vi "Dashboard Main.vi"() -> ()   [LabVIEW 2012]
uses:
  Sally_Framework_2013/AutoEnum.ctl
  Sally_Framework_2013/LauncherPresets.ctl
  Sally_Framework_2013/AutoInstructArray.ctl
  Sally_Framework_2013/AutoInstruction.ctl
  <vilib>/event_ctls.llb/eventvkey.ctl
  DBNameEnum.ctl
  <vilib>/Utility/config.llb/Read Key (String).vi
  <vilib>/Utility/config.llb/Read Key (I32).vi
  <vilib>/Utility/config.llb/Write Key (String).vi
  <vilib>/Utility/config.llb/Write Key (I32).vi
  <vilib>/Utility/config.llb/NI_LVConfig.lvlib
panel:
  out "Battery Value":dbl(slide) scale=0.0..14.0 scale format="%#_2e"
  out "Battery":sgl(graph)
  in  "Camera Settings":T1={"Frate Rate"=30, "Compression"=30, "Size"=1} {"Frate Rate" scale=1.0..30.0; "Size" items=["640x480", "320x240", "160x120"]}
  out "Mode":T2(ring)=enum."Auto Disabled"
  out "Camera IP":string
  out "Robot IP":string
  in  "Dashboard Tab":T3(tab)
  out "ReverseDrive":bool
  in  "Use2DriveAlign":bool=TRUE
  out "DriveAlignLSRight":bool
  out "ClimbLS":bool
  in  "UseLauncherPID":bool=TRUE
  in  "UseAngleEncoder":bool=TRUE
  in  "UseLauncherEncoder":bool=TRUE
  out "LauncherAngleMatches":bool
  out "sDriveDistance":dbl
  out "Drive Loop Timing (ms)":u32
  in  "AutoEnum":T4=enum."BehindPyramid"
  out "LauncherMotorValue":dbl
  out "Version":string
  out "LauncherAngle":cluster{dbl, dbl}(knob) scale=0.0..55.0 scale format="%#2_3g"
  out "DriveAlignLSLeft":bool
  out "LauncherRPM":cluster{dbl, dbl}(knob) scale=0.0..4000.0
  in  "Disabled":T5=[{"Distance/Angle"=10.0, "Speed"=0.0, "Action"=enum."Wait", "NumFrisbees"=0}]
  in  "BehindPyramid":T5=[{"Distance/Angle"=30.0, "Speed"=2390.0, "Action"=enum."Aim", "NumFrisbees"=0}, {"Distance/Angle"=5.0, "Speed"=0.0, "Action"=enum."Wait", "NumFrisbees"=0}, {"Distance/Angle"=0.0, "Speed"=0.0, "Action"=enum."Shoot", "NumFrisbees"=4}]
  in  "CloseLeft":T5=[{"Distance/Angle"=34.0, "Speed"=2390.0, "Action"=enum."Aim", "NumFrisbees"=0}, {"Distance/Angle"=5.0, "Speed"=0.0, "Action"=enum."Wait", "NumFrisbees"=0}, {"Distance/Angle"=0.0, "Speed"=0.0, "Action"=enum."Shoot", "NumFrisbees"=4}]
  in  "CloseRight":T5=[{"Distance/Angle"=34.0, "Speed"=2390.0, "Action"=enum."Aim", "NumFrisbees"=0}, {"Distance/Angle"=5.0, "Speed"=0.0, "Action"=enum."Wait", "NumFrisbees"=0}, {"Distance/Angle"=0.0, "Speed"=0.0, "Action"=enum."Shoot", "NumFrisbees"=4}]
  in  "BackLeft":T5=[{"Distance/Angle"=29.0, "Speed"=2390.0, "Action"=enum."Aim", "NumFrisbees"=0}, {"Distance/Angle"=5.0, "Speed"=0.0, "Action"=enum."Wait", "NumFrisbees"=0}, {"Distance/Angle"=0.0, "Speed"=0.0, "Action"=enum."Shoot", "NumFrisbees"=4}]
  in  "BackRight":T5=[{"Distance/Angle"=29.0, "Speed"=2390.0, "Action"=enum."Aim", "NumFrisbees"=0}, {"Distance/Angle"=5.0, "Speed"=0.0, "Action"=enum."Wait", "NumFrisbees"=0}, {"Distance/Angle"=0.0, "Speed"=0.0, "Action"=enum."Shoot", "NumFrisbees"=4}]
  in  "BackupAuto":dbl[](array[numeric])=[2390.0, 30.0, 3.0, 4.0, 2000.0, -0.5]
  in  "UseClusterArray":bool
  in  "PullbackTol":dbl=100.0
  in  "FireTol":dbl=10.0
  in  "LauncherRPMTol":dbl=10.0
  in  "LauncherAngleTol":dbl=0.1
  in  "InitialWait (ms)":dbl=5000.0
  in  "WaitBetweenLaunch (ms)":dbl=1200.0
  in  "QSWaitBeforeFire (ms)":dbl=600.0
  in  "QSWaitBeforeRetract (ms)":dbl=100.0
  in  "AngleForwardValue":dbl=0.8
  in  "AngleBackwardValue":dbl=-0.8
  in  "HalfSpeedFactor":dbl=0.75
  in  "RPMPresets":T7={"cPresetPyramid"=2390.0, "cPresetShort"=2390.0, "cPresetMid"=1950.0, "cPresetFar"=2390.0, "cPresetClimbHigh"=0.0, "cPresetClimbLow"=0.0}
  in  "AnglePresets":T7={"cPresetPyramid"=30.0, "cPresetShort"=50.0, "cPresetMid"=51.5, "cPresetFar"=25.0, "cPresetClimbHigh"=32.0, "cPresetClimbLow"=20.0}
  in  "Slider":dbl(slide) scale=0.0..100.0 scale format="%#_3g"
  in  "On/Off":bool caption="Solenoid"
  in  "Test Name":u16(ring) items=["Select the test to run...", "Example Test", "-------------------------------", "List of tests is built in robot code.", "Replace with your own automated tests."]
  in  "Test Tree":string(tree)
  in  "Motor":cluster{"Value":dbl, "Enable":bool} {"Value" scale=-1.0..1.0 scale format="%#_3g"}
  out "Progress":T8 {"Test Progress" scale=0.0..100.0}
  in  "Rev/Fwd":cluster{"Forward":bool, "Reverse":bool}
  in  "Ring":u16(ring) items=["Auto", "Fixed indoor", "Fixed outdoor 1", "Fixed outdoor 2", "Fixed fluorescent 1", "Fixed fluorescent 2", "Hold current"]
  in  "Listbox":i32(listbox)=8
  in  "Viewer":T9(tab)
  out "Mbps":dbl format="%#.1g"
  in  "Enable":bool=TRUE
  in  "DB Camera Config":bool
  out "Mbps":bool
  out "fps":dbl format="%#.1g"
  out "Image Error Message":string="Timeout in Camera Communications"
  out "Camera Image":T10(plugin-control)
  out "Buttons 1":cluster{"1":bool, "2":bool, "3":bool}
  out "Kinect 1":cluster{"X":dbl, "Y":dbl, "Z":dbl} {"X" scale=1.0..-1.0; "Y" scale=1.0..-1.0; "Z" scale=1.0..-1.0}
  out "Buttons 2":cluster{"1":bool, "2":bool, "3":bool}
  out "Kinect 2":cluster{"X":dbl, "Y":dbl, "Z":dbl} {"X" scale=1.0..-1.0; "Y" scale=1.0..-1.0; "Z" scale=1.0..-1.0}
  out "Version":string
  out "Skeleton Picture":picture
  out "Players":i8
  out "Tree":string(tree)
  # "Drive & Motors"
  # "Robot IP:"
  # "sLauncherRPM"
  # "TargetLauncherRPM"
  # "sLauncherAngle"
  # "LauncherTargetAngle"
  # "RPM"
  # "Angle"
  # "Wait (s)"
  # "ShootNum"
  # "Time (ms)"
  # "Motor Value"
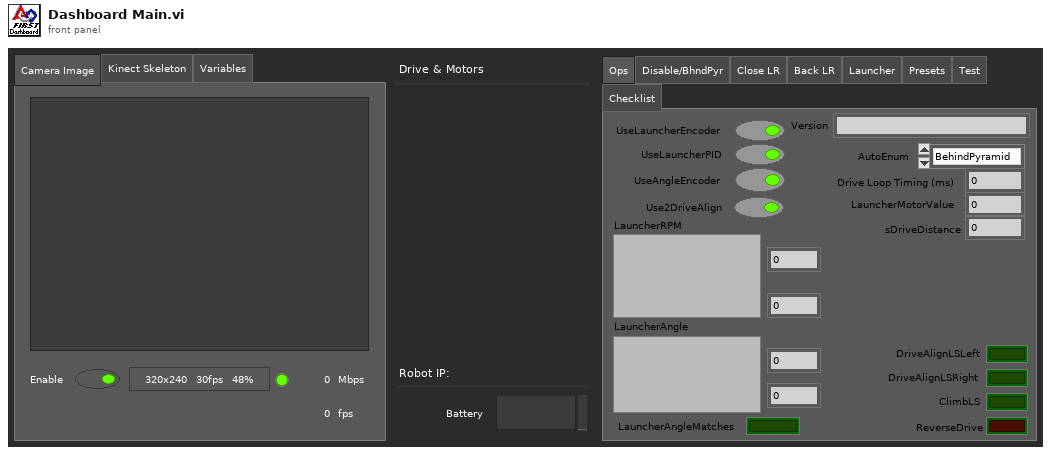
[diagram p1: front panel]
types:
  T1 = cluster{"Frate Rate":i32, "Compression":i32, "Size":u16}
  T2 = enum8{"Tele-Op Disabled", "Tele-Op Enabled", "Auto Disabled", "Auto Enabled", "Test Disabled", "Test Enabled", ""}
  T3 = enum32{"Ops", "Disable/BhndPyr", "Close LR", "Back LR", "Launcher", "Presets", "Test", "Checklist"}
  T4 = typedef "AutoEnum.ctl" = enum16{"Disabled", "BackRight", "BackLeft", "CloseRight", "CloseLeft", "BehindPyramid"}
  T5 = typedef "AutoInstructArray.ctl" = T6[]
  T6 = typedef "AutoInstruction.ctl" = cluster{"Distance/Angle":dbl, "Speed":dbl, "Action":enum16{"DriveForward", "Turn", "Aim", "Shoot", "Wait"}, "NumFrisbees":i32}
  T7 = typedef "LauncherPresets.ctl" = cluster{"cPresetPyramid":dbl, "cPresetShort":dbl, "cPresetMid":dbl, "cPresetFar":dbl, "cPresetClimbHigh":dbl, "cPresetClimbLow":dbl}
  T8 = cluster{"Test Progress":u8, "Test Progress Text":string}
  T9 = enum32{"Camera Image", "Kinect Skeleton", "Variables"}
  T10 = typedef "IMAQ Image.ctl" = refnum<image>
  T11 = typedef "Image Type" = u32
  T12 = typedef "LVBoundsTypeDef.ctl" = cluster{"Width":u32, "Height":u32}
  T13 = typedef "SkeletonTrackState.ctl" = enum32{"NotTracked", "PositionOnly", "Tracked"}
  T14 = cluster{"TrackingState":u8[], "Position":cluster{"x":sgl, "y":sgl, "z":sgl}, cluster{"x":sgl, "y":sgl, "z":sgl, sgl}[], "TrackState":T13}
  T15 = cluster{cluster{"ScaledToPercentRange":dbl, "ScaledToPercentRange":dbl, "ScaledToPercentRange":dbl}, cluster{bool, bool, bool}}[]
  T16 = cluster{cluster{"ScaledToPercentRange":dbl, "ScaledToPercentRange":dbl, "ScaledToPercentRange":dbl}, cluster{bool, bool, bool}}
  T17 = cluster{"ScaledToPercentRange":dbl, "ScaledToPercentRange":dbl, "ScaledToPercentRange":dbl}
  T18 = typedef "LVRectTypeDef.ctl" = cluster{"Left":i16, "Top":i16, "Right":i16, "Bottom":i16}
  T19 = typedef "DBNameEnum.ctl" = enum16{"AutoInstructions", "DriveLoopTime", "DriveAlignLSLeft", "DriveAlignLSRight", "Use2DriveAlign", "ClimbLS", "LauncherAngleMatches", "FrameworkVersion", "sLauncherAngle", "LauncherTargetAngle", "sLauncherRPM", "LauncherTargetRPM", "sDriveDistance", "LauncherMotorValue", "PullbackTol", "FireTol", "LauncherRPMTol", "LauncherAngleTol", "InitialWait", "WaitBetweenLaunch", "AnglePresets", "RPMPresets", "UseAngleEncoder", "UseLauncherEncoder", "UseLauncherPID", "QSWaitBeforeFire", "QSWaitBeforeRetract", "AngleForwardValue", "AngleBackwardValue", "UseClusterArray", "BackupAuto", "ReverseDriveIndicate", "HalfSpeedFactor"}
  T20 = cluster{"Competition mode":bool, "Robot Link":bool, "Autonomous":bool, "Enabled":bool, "E-Stop":bool, "Simulated":bool, "TestMode":bool, "Docked Window":bool}
  T21 = typedef "NI_LVConfig.lvlib/Config Data RefNum.ctl" = refnum<k1>
  T22 = typedef "eventvkey.ctl" = enum16{"ASCII", "Enter", "Return", "Shift", "Ctrl", "Alt", "Cmd", "Opt", "Caps", "NumLock", "Clear", "Break", "Up", "Down", "Left", "Right", "Insert", "Delete", "Home", "End", "PageUp", "PageDown", "Escape", "Help", "Pause", "ScrollLock", "F1", "F2", "F3", "F4", "F5", "F6", "F7", "F8", "F9", "F10", "F11", "F12", "F13", "F14", "F15", "F16", "F17", "F18", "F19", "F20", "F21", "F22", "F23", "F24", "Play", "VolumeUp", "VolumeDown", "Mute", "Two Byte Char"}
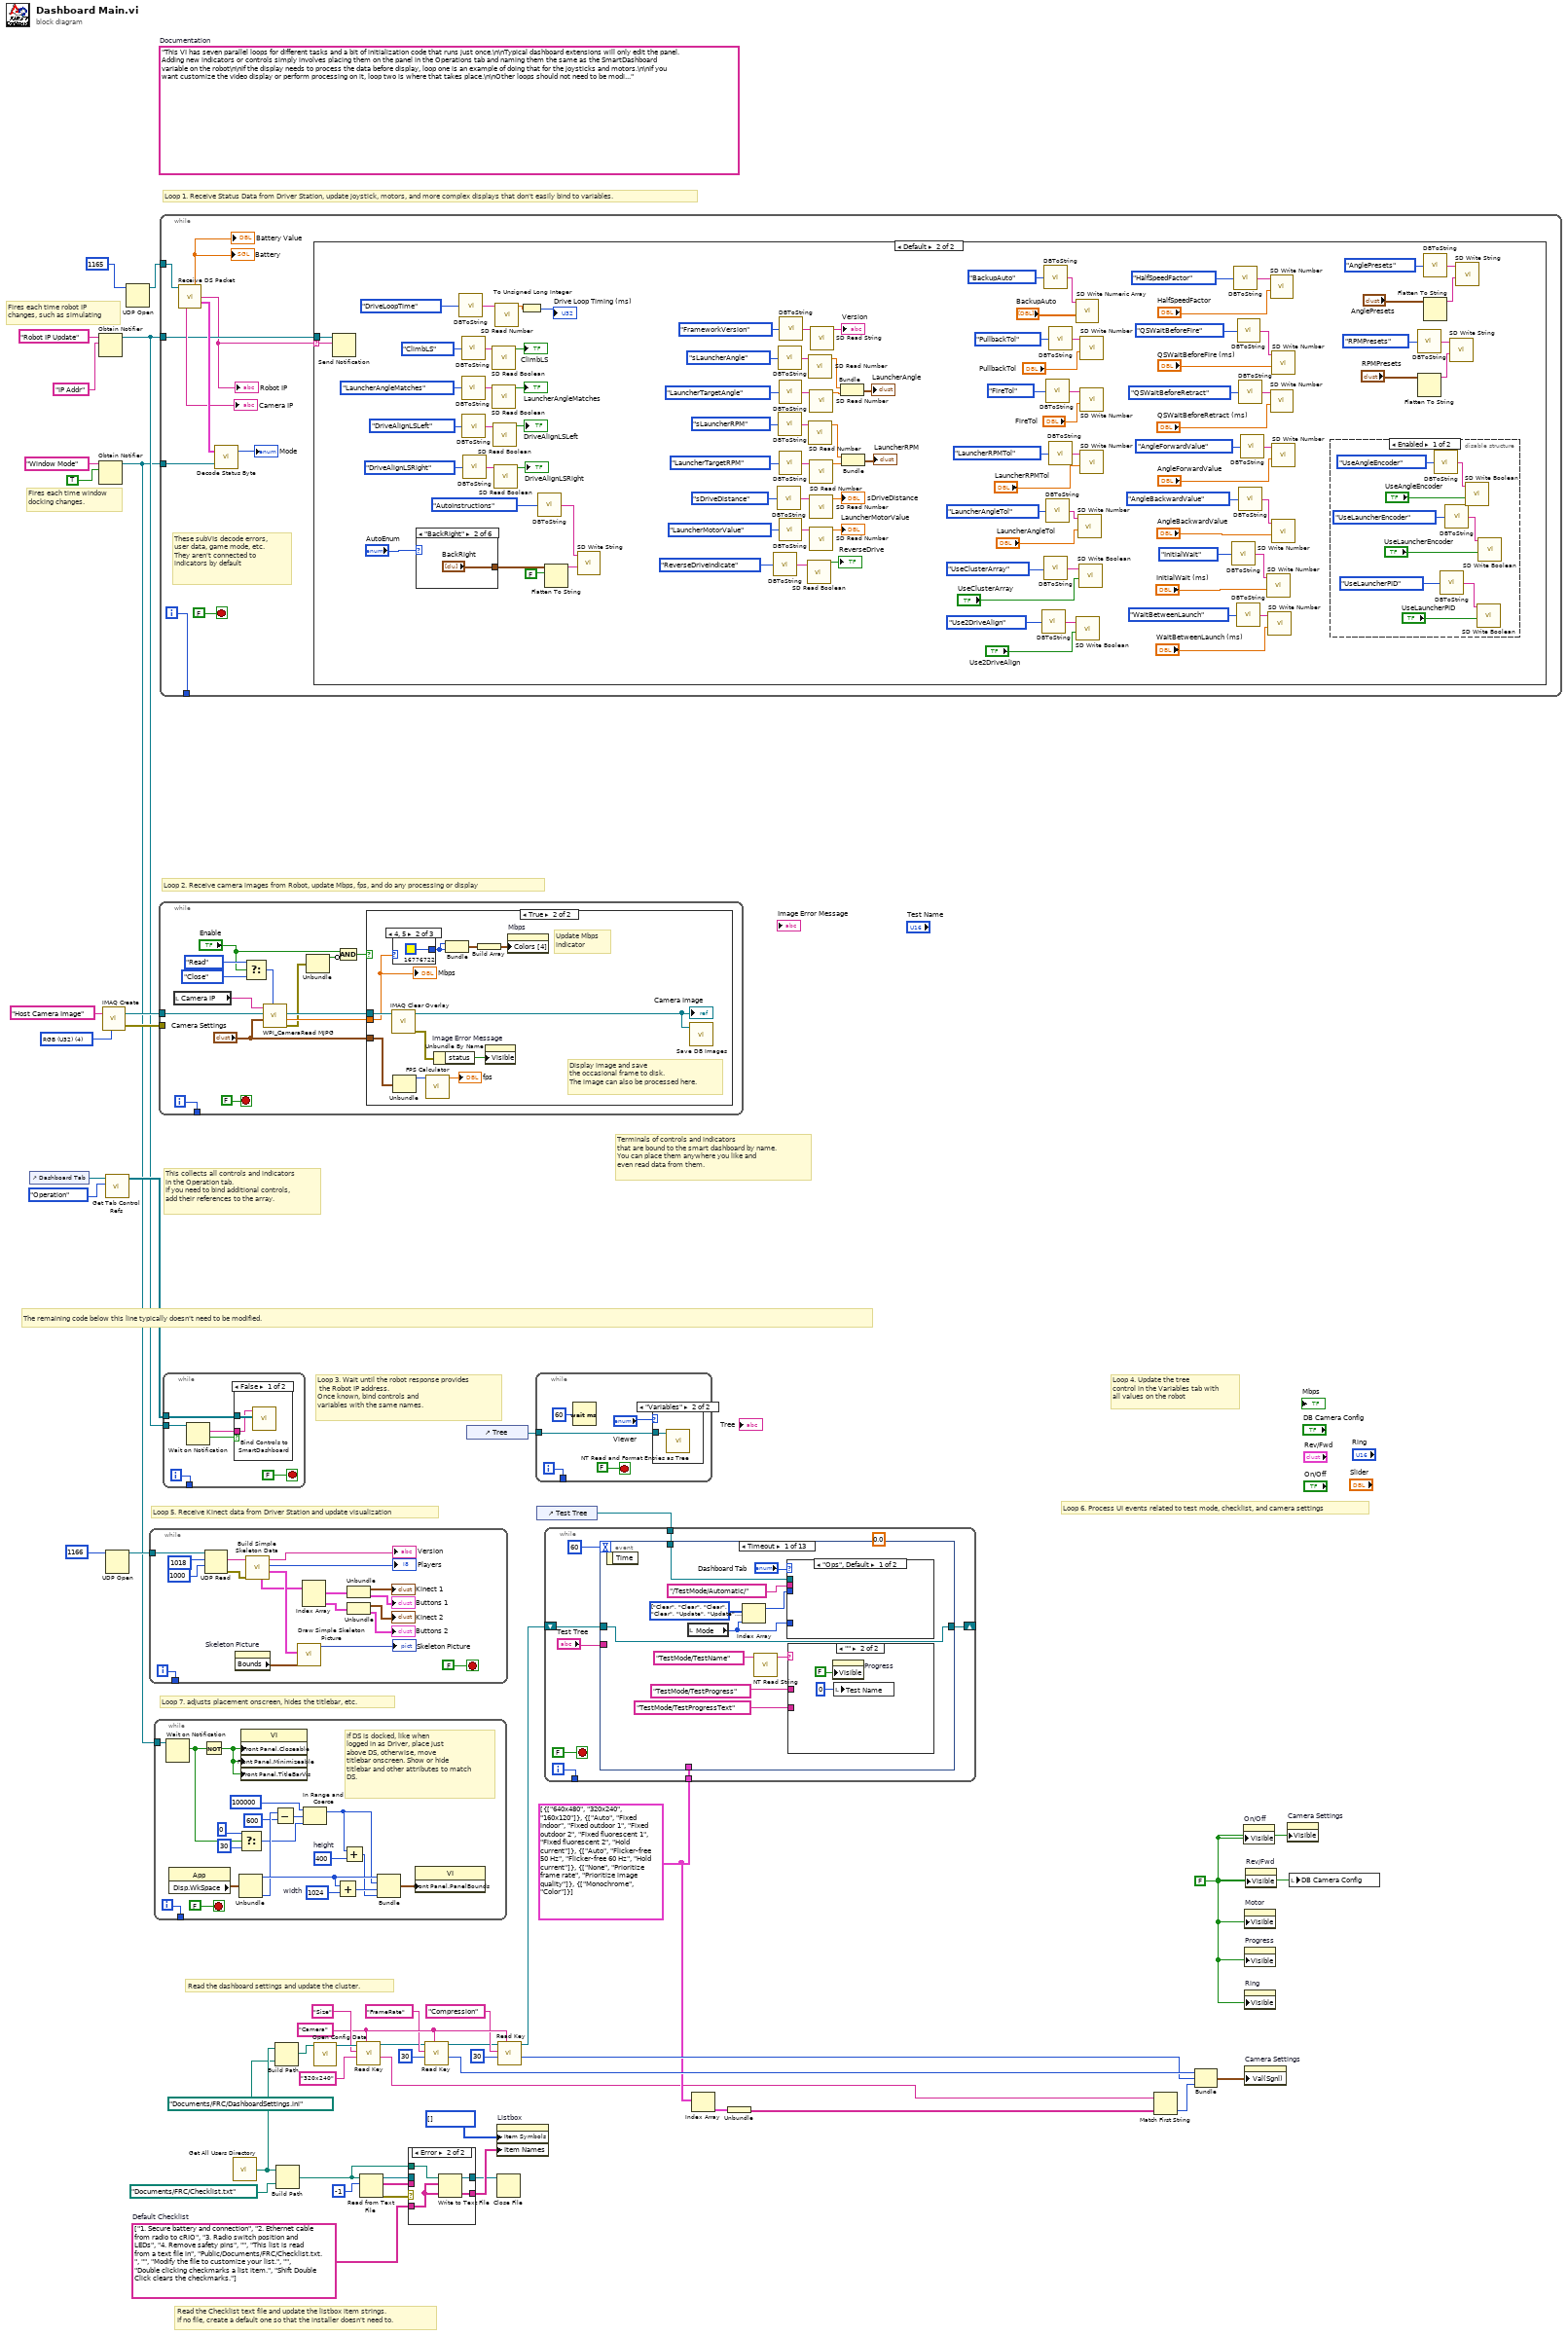
[diagram p0: block diagram]
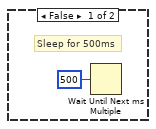
[diagram p3: hidden frame]
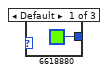
[diagram p4: hidden frame]
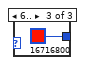
[diagram p5: hidden frame]
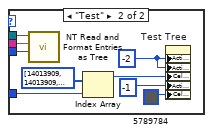
[diagram p7: hidden frame]
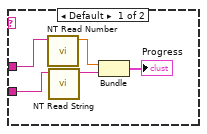
[diagram p8: hidden frame]
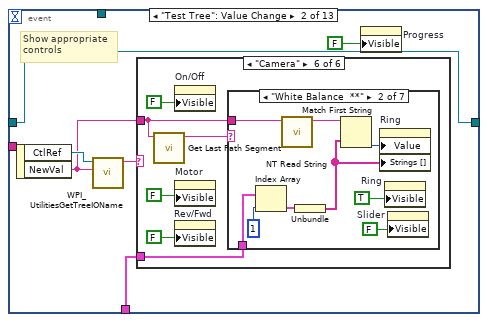
[diagram p9: hidden frame]
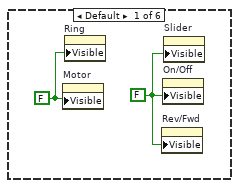
[diagram p10: hidden frame]
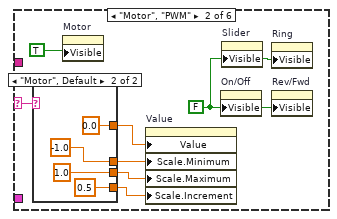
[diagram p11: hidden frame]
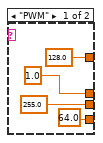
[diagram p12: hidden frame]
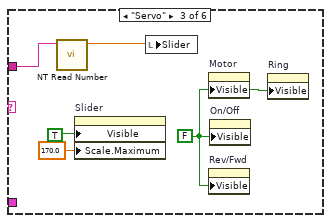
[diagram p13: hidden frame]
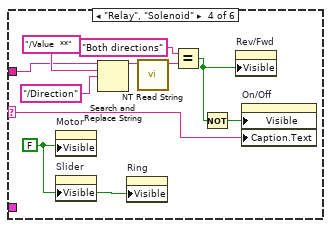
[diagram p14: hidden frame]
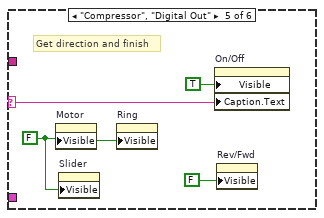
[diagram p15: hidden frame]
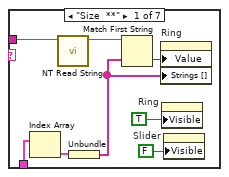
[diagram p16: hidden frame]
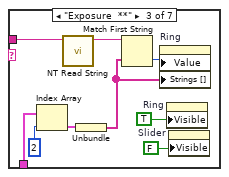
[diagram p17: hidden frame]
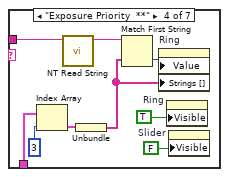
[diagram p18: hidden frame]
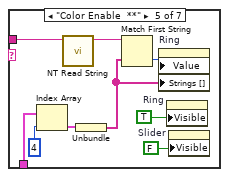
[diagram p19: hidden frame]
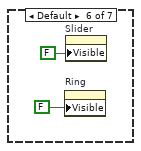
[diagram p20: hidden frame]
diagram:
  w21 = "Camera"
  w13 = cluster{string[]}[] [{["640x480", "320x240", "160x120"]}, {["Auto", "Fixed indoor", "Fixed outdoor 1", "Fixed outdoor 2", "Fixed fluorescent 1", "Fixed fluorescent 2", "Hold current"]}, {["Auto", "Flicker-free 50 Hz", "Flicker-free 60 Hz", "Hold current"]}, {["None", "Prioritize frame rate", "Prioritize image quality"]}, {["Monochrome", "Color"]}]
  w29 = string[] ["1. Secure battery and connection", "2. Ethernet cable from radio to cRIO", "3. Radio switch position and LEDs", "4. Remove safety pins", "", "This list is read from a text file in", "Public/Documents/FRC/Checklist.txt.", "", "Modify the file to customize your list.", "", "Double clicking checkmarks a list item.", "Shift Double Click clears the checkmarks."]  # Default Checklist
  w27 = FALSE ("Visible")
  (unwired) "This VI has seven parallel loops for different tasks and a bit of initialization code that runs just once.\n\nTypical dashboard extensions will only edit the panel. Adding new indicators or controls simply involves placing them on the panel in the Operations tab and naming them the same as the SmartDashboard variable on the robot\n\nIf the display needs to process the data before display, loop one is an example of doing that for the joysticks and motors.\n\nIf you want customize the video display or perform processing on it, loop two is where that takes place.\n\nOther loops should not need to be modified. They are pretty standard, and document the task they perform."  # Documentation
  w50 = T11 4 items=["Grayscale (U8)", "Grayscale (I16)", "Grayscale (SGL)", "Complex (CSG)", "RGB (U32)", "HSL (U32)", "RGB (U64)"] ("Image Type")
  # "Fires each time robot IP\nchanges, such as simulating"
  # "Fires each time window\ndocking changes."
  # "Read the Checklist text file and update the listbox item strings.\nIf no file, create a default one so that the installer doesn't need to."
  # "This collects all controls and indicators\nin the Operation tab.\nIf you need to bind additional controls,\nadd their references to the array."
  # "The remaining code below this line typically doesn't need to be modified."
  # "Loop 6. Process UI events related to test mode, checklist, and camera settings"
  # "Read the dashboard settings and update the cluster."
  # "Terminals of controls and indicators\nthat are bound to the smart dashboard by name.\nYou can place them anywhere you like and\neven read data from them."
  # "Loop 4. Update the tree\ncontrol in the Variables tab with\nall values on the robot"
  # "Loop 3. Wait until the robot response provides\n the Robot IP address.\nOnce known, bind controls and\nvariables with the same names."
  # "Loop 5. Receive Kinect data from Driver Station and update visualization"
  # "Loop 7. adjusts placement onscreen, hides the titlebar, etc."
  # "Loop 1. Receive Status Data from Driver Station, update joystick, motors, and more complex displays that don't easily bind to variables."
  # "Loop 2. Receive camera images from Robot, update Mbps, fps, and do any processing or display"
  n1 = control-ref of="Dashboard Tab"() -> (w43:refnum<vi>)
  n2 = Obtain Notifier(name (unnamed)="Robot IP Update", notification data type="IP Addr" ("name (unnamed)")) -> (notifier out=w40:refnum<notifier>)  [unwired: 2 in, 2 out]
  n3 = Obtain Notifier(name (unnamed)="Window Mode", notification data type=TRUE) -> (notifier out=w33:refnum<notifier>)  [unwired: 2 in, 2 out]
  n4 = call "IMAQ Create"("Image Name"="Host Camera Image", "Image Type"=w50) -> ("New Image"=w48:T10, "error out"=w47:errorcluster)  [unwired: 2 in, 1 out]
  n5 = call <vilib>:"Get Tab Control Refs.vi"("Page Index"=enum32{"Operation", "Test"}."Operation" ("Dashboard Tab"), "TabControl in"=w43) -> ("ControlsOnPage"=w44:refnum<vi>[])  [unwired: 9 in]
  n6 = UDP Open(11:u16 1166 ("port")) -> (port=w45:refnum<k16>)  [unwired: 2 in, 4 out]
  n7 = UDP Open(11:u16 1165 ("port")) -> (port=w51:refnum<k16>)  [unwired: 2 in, 4 out]
  n8 = while {
    tunnel: w45 -> [w69]
    tunnel: [w54] -> _
    i -> [w54]
    stop <- FALSE stop-if-true
    n9 = UDP Read(connection ID=w69, max size (548)=1018 ("bytes to read"), timeout ms (25000)=1000) -> (data out=w63:string, error out=w53:errorcluster)  [unwired: 1 in, 3 out]
    n10 = property on="Skeleton Picture" class="Pict"() -> ("Bounds"=w65:T12)  [unwired: 2 in, 2 out]
    n11 = call "Build Simple Skeleton Data.vi"("error in (no error)"=w53, "data in"=w63) -> ("Skeleton Data"=w64:T14, "NumPlayers"=→"Players":i8, "Version String"=→"Version":string, "Simple Joystick Info"=w61:T15)  [unwired: 5 in, 1 out]
    n12 = call "Draw Simple Skeleton Picture.vi"("Bounds"=w65, "Simple Skeleton"=w64) -> ("new picture out"=→"Skeleton Picture":picture)  [unwired: 9 in]
    n13 = Index Array(array=w61) -> (element #1=w60:T16, element #2=w59:T16)  [unwired: 2 in]
    n14 = Unbundle(w60) -> (→"Kinect 1":T17, →"Buttons 1":cluster{bool, bool, bool})
    n15 = Unbundle(w59) -> (→"Kinect 2":T17, →"Buttons 2":cluster{bool, bool, bool})
  }
  n16 = while {
    tunnel: w33 -> [w90]
    tunnel: [w88] -> _
    i -> [w88]
    stop <- FALSE stop-if-true
    w80 = 1024  # width
    w83 = 400  # height
    # "If DS is docked, like when\nlogged in as Driver, place just\nabove DS, otherwise, move\ntitlebar onscreen. Show or hide\ntitlebar and other attributes to match\nDS."
    n17 = Wait on Notification(notifier=w90) -> (notification=w75:bool)  [unwired: 3 in, 3 out]
    n18 = property class="App"() -> ("Disp.WkSpace"=w86:T18)  [unwired: 2 in, 2 out]
    n19 = Not(x=w75) -> (.not. x?=w89:bool)
    n20 = Unbundle(w86) -> ("Left"=w84:i16, "Bottom"=w81:i16)  [unwired: 2 out]
    n21 = Select(t=0, s=w75, f=30) -> (s? t:f=w74:i32)
    n22 = property class="VI"("Front Panel.Closeable"=w89, "Front Panel.Minimizeable"=w89, "Front Panel.TitleBarVis"=w89) -> ()  [unwired: 2 in, 2 out]
    n23 = Subtract(x=w81, y=600) -> (x-y=w78:i32)
    n24 = In Range and Coerce(upper limit=100000, x=w78, lower limit=w74) -> (coerced(x)=w72:i32)  [unwired: 1 out]
    n25 = Add(x=w84, y=w80) -> (x+y=w85:i32)
    n26 = Add(x=w72, y=w83) -> (x+y=w82:i32)
    n27 = Bundle("Left"=w84, w72, w85, w82) -> (w87:cluster{"Left":i16, i32, i32, i32})  [unwired: 1 out]
    n28 = property class="VI"("Front Panel.PanelBounds"=w87) -> ()  [unwired: 2 in, 2 out]
  }
  n29 = while {
    tunnel: w48 -> [w101]
    tunnel: w47 -> [_]
    tunnel: [w104] -> _
    i -> [w104]
    stop <- FALSE stop-if-true
    n30 = local read "Camera IP"() -> (w103:string)
    n31 = Select(t=enum16{"Read", "Reopen", "Close"}."Read" ("Operation"), s="Enable", f=enum16{"Read", "Reopen", "Close"}."Close" ("Operation")) -> (s? t:f=w96:enum16{"Read", "Reopen", "Close"})
    n32 = call <vilib>:"WPI_CameraRead MJPG.vi"("Operation"=w96, "Camera Settings"="Camera Settings", "Image"=w101, "address"=w103) -> ("error out"=w95:errorcluster, "Bandwidth (kbps)"=w99:dbl, "Image Out"=w100:T10)  [unwired: 5 in]
    n33 = Unbundle(w95) -> ("status"=w93:bool)  [unwired: 2 out]
    n34 = Compound Arithmetic op=AND("Enable", invert w93) -> (w92:bool)
    n35 = case shown="True" w92 {
      tunnel: "Camera Settings" -> [_ w108]
      tunnel: w100 -> [_ w111]
      tunnel: w99 -> [_ w110]
      frame False {
        # "Sleep for 500ms"
        n36 = Wait Until Next ms Multiple(millisecond multiple=u32 500) -> ()  [unwired: 1 out]
      }
      frame True {
        # "Display image and save\nthe occasional frame to disk.\nThe image can also be processed here."
        # "Update Mbps\nindicator"
        n37 = call "IMAQ Clear Overlay"("Image"=w111) -> ("error out"=w116:errorcluster, "Image Out"=w115:T10)  [unwired: 2 in, 7 out]
        "Camera Image" <- w115
        n38 = case shown="4, 5" w110 {
          tunnel: [u32 6618880 ("Color Box") u32 16776722 ("Color Box") u32 16716800 ("Color Box")] -> w112
          frame Default {
          }
          frame 4, 5 {
          }
          frame 6.. {
          }
        }
        n39 = Unbundle(w108) -> ("Frate Rate"=w107:i32)  [unwired: 2 out]
        n40 = call "FPS Calculator.vi"("Average Count"=w107) -> ("fps"=→"fps":dbl)  [unwired: 10 in]
        n41 = Unbundle By Name(w116) -> ("status"=w117:bool)
        n42 = Bundle("Color Box"=w112, "Color Box"=w112) -> (w114:cluster{"Color Box":u32, "Color Box":u32})  [unwired: 1 out]
        n43 = Build Array(w114) -> (w113:cluster{"Color Box":u32, "Color Box":u32}[])
        n44 = property on="Image Error Message" class="Str"("Visible"=w117) -> ()  [unwired: 2 in, 2 out]
        n45 = property on="Mbps" class="Bool (strict)"("Colors [4]"=w113) -> ()  [unwired: 2 in, 2 out]
        n46 = call "Save DB Images.vi"("Image"=w115) -> ()  [unwired: 2 in, 1 out]
        "Mbps" <- w110
      }
    }
  }
  n47 = while {
    tunnel: w51 -> [w128]
    tunnel: w40 -> [w122]
    tunnel: w33 -> [w126]
    tunnel: [w123] -> _
    i -> [w123]
    stop <- FALSE stop-if-true
    # "These subVIs decode errors, user data, game mode, etc.\nThey aren't connected to indicators by default"
    n48 = call "Receive DS Packet.vi"("Recv Socket"=w128) -> ("Battery"=→"Battery" →"Battery Value":sgl, "Robot IP Address"=w121:string, "Status"=w129:T20, "Camera IP Address"=→"Camera IP":string)  [unwired: 1 in, 10 out]
    "Robot IP" <- w121
    n49 = call "Decode Status Byte.vi"("Window Mode Notifier"=w126, "Status"=w129) -> ("Mode"=→"Mode":T2)  [unwired: 1 out]
    n50 = case shown="Default" w121 {
      selector: w121 -> [_ w229]
      tunnel: w122 -> [_ w230]
      frame "0.0.0.0" {
        # "Robot not responding, don't poll the variables"
      }
      frame Default {
        n51 = Send Notification(notification=w229, notifier=w230) -> ()  [unwired: 1 in, 2 out]
        n52 = case shown="\"BackRight\"" "AutoEnum" {
          tunnel: ["Disabled" "BackRight" "BackLeft" "CloseRight" "CloseLeft" "BehindPyramid"] -> w164
          frame "Disabled" {
          }
          frame "BackRight" {
          }
          frame "BackLeft" {
          }
          frame "CloseRight" {
          }
          frame "CloseLeft" {
          }
          frame "BehindPyramid", Default {
          }
        }
        n53 = call "DBToString.vi"("Enum"=DBNameEnum."DriveLoopTime") -> ("Refname"=w162:string)
        n54 = call "DBToString.vi"("Enum"=DBNameEnum."ClimbLS") -> ("Refname"=w170:string)
        n55 = call "DBToString.vi"("Enum"=DBNameEnum."LauncherAngleMatches") -> ("Refname"=w169:string)
        n56 = call "DBToString.vi"("Enum"=DBNameEnum."DriveAlignLSLeft") -> ("Refname"=w173:string)
        n57 = call "DBToString.vi"("Enum"=DBNameEnum."DriveAlignLSRight") -> ("Refname"=w161:string)
        n58 = call <vilib>:"SD Read Boolean.vi"("Name"=w170) -> ("Boolean"=→"ClimbLS":bool)  [unwired: 8 in, 2 out]
        n59 = call <vilib>:"SD Read Boolean.vi"("Name"=w169) -> ("Boolean"=→"LauncherAngleMatches":bool)  [unwired: 8 in, 2 out]
        n60 = call <vilib>:"SD Read Boolean.vi"("Name"=w173) -> ("Boolean"=→"DriveAlignLSLeft":bool)  [unwired: 8 in, 2 out]
        n61 = call <vilib>:"SD Read Boolean.vi"("Name"=w161) -> ("Boolean"=→"DriveAlignLSRight":bool)  [unwired: 8 in, 2 out]
        n62 = call <vilib>:"SD Read Number.vi"("Name"=w162) -> ("Numeric"=w228:dbl)  [unwired: 8 in, 2 out]
        n63 = To Unsigned Long Integer(number=w228) -> (unsigned 32bit integer=→"Drive Loop Timing (ms)":u32)
        n64 = call "DBToString.vi"("Enum"=DBNameEnum."AutoInstructions") -> ("Refname"=w167:string)
        n65 = Flatten To String(anything=w164, prepend array or string size? (T)=FALSE) -> (data string=w165:string)  [unwired: 2 in, 2 out]
        n66 = call <vilib>:"SD Write String.vi"("String"=w165, "Name"=w167) -> ()  [unwired: 8 in, 2 out]
        n67 = call "DBToString.vi"("Enum"=DBNameEnum."ReverseDriveIndicate") -> ("Refname"=w134:string)
        n68 = call "DBToString.vi"("Enum"=DBNameEnum."sDriveDistance") -> ("Refname"=w175:string)
        n69 = call "DBToString.vi"("Enum"=DBNameEnum."sLauncherAngle") -> ("Refname"=w181:string)
        n70 = call "DBToString.vi"("Enum"=DBNameEnum."sLauncherRPM") -> ("Refname"=w179:string)
        n71 = call "DBToString.vi"("Enum"=DBNameEnum."LauncherTargetAngle") -> ("Refname"=w180:string)
        n72 = call "DBToString.vi"("Enum"=DBNameEnum."LauncherTargetRPM") -> ("Refname"=w178:string)
        n73 = call "DBToString.vi"("Enum"=DBNameEnum."LauncherMotorValue") -> ("Refname"=w187:string)
        n74 = call "DBToString.vi"("Enum"=DBNameEnum."FrameworkVersion") -> ("Refname"=w177:string)
        n75 = call <vilib>:"SD Read Boolean.vi"("Name"=w134) -> ("Boolean"=→"ReverseDrive":bool)  [unwired: 8 in, 2 out]
        n76 = call <vilib>:"SD Read Number.vi"("Name"=w181) -> ("Numeric"=w214:dbl)  [unwired: 8 in, 2 out]
        n77 = call <vilib>:"SD Read Number.vi"("Name"=w179) -> ("Numeric"=w210:dbl)  [unwired: 8 in, 2 out]
        n78 = call <vilib>:"SD Read Number.vi"("Name"=w180) -> ("Numeric"=w215:dbl)  [unwired: 8 in, 2 out]
        n79 = call <vilib>:"SD Read Number.vi"("Name"=w178) -> ("Numeric"=w211:dbl)  [unwired: 8 in, 2 out]
        n80 = call <vilib>:"SD Read Number.vi"("Name"=w175) -> ("Numeric"=→"sDriveDistance":dbl)  [unwired: 8 in, 2 out]
        n81 = call <vilib>:"SD Read Number.vi"("Name"=w187) -> ("Numeric"=→"LauncherMotorValue":dbl)  [unwired: 8 in, 2 out]
        n82 = call <vilib>:"SD Read String.vi"("Name"=w177) -> ("String"=→"Version":string)  [unwired: 8 in, 2 out]
        n83 = Bundle("Numeric"=w214, "Numeric"=w215) -> (→"LauncherAngle":cluster{"Numeric":dbl, "Numeric":dbl})  [unwired: 1 in]
        n84 = Bundle("Numeric"=w210, "Numeric"=w211) -> (→"LauncherRPM":cluster{"Numeric":dbl, "Numeric":dbl})  [unwired: 1 in]
        n85 = call "DBToString.vi"("Enum"=DBNameEnum."Use2DriveAlign") -> ("Refname"=w157:string)
        n86 = call "DBToString.vi"("Enum"=DBNameEnum."BackupAuto") -> ("Refname"=w139:string)
        n87 = call "DBToString.vi"("Enum"=DBNameEnum."UseClusterArray") -> ("Refname"=w142:string)
        n88 = call "DBToString.vi"("Enum"=DBNameEnum."FireTol") -> ("Refname"=w189:string)
        n89 = call "DBToString.vi"("Enum"=DBNameEnum."LauncherAngleTol") -> ("Refname"=w191:string)
        n90 = call "DBToString.vi"("Enum"=DBNameEnum."PullbackTol") -> ("Refname"=w188:string)
        n91 = call "DBToString.vi"("Enum"=DBNameEnum."LauncherRPMTol") -> ("Refname"=w190:string)
        n92 = call <vilib>:"SD Write Numeric Array.vi"("Numeric Array"="BackupAuto", "Name"=w139) -> ()  [unwired: 8 in, 2 out]
        n93 = call <vilib>:"SD Write Boolean.vi"("Boolean"="Use2DriveAlign", "Name"=w157) -> ()  [unwired: 8 in, 2 out]
        n94 = call <vilib>:"SD Write Number.vi"("Numeric"="LauncherAngleTol", "Name"=w191) -> ()  [unwired: 8 in, 2 out]
        n95 = call <vilib>:"SD Write Boolean.vi"("Boolean"="UseClusterArray", "Name"=w142) -> ()  [unwired: 8 in, 2 out]
        n96 = call <vilib>:"SD Write Number.vi"("Numeric"="PullbackTol", "Name"=w188) -> ()  [unwired: 8 in, 2 out]
        n97 = call <vilib>:"SD Write Number.vi"("Numeric"="FireTol", "Name"=w189) -> ()  [unwired: 8 in, 2 out]
        n98 = call <vilib>:"SD Write Number.vi"("Numeric"="LauncherRPMTol", "Name"=w190) -> ()  [unwired: 8 in, 2 out]
        n99 = call "DBToString.vi"("Enum"=DBNameEnum."InitialWait") -> ("Refname"=w203:string)
        n100 = call "DBToString.vi"("Enum"=DBNameEnum."HalfSpeedFactor") -> ("Refname"=w131:string)
        n101 = call "DBToString.vi"("Enum"=DBNameEnum."WaitBetweenLaunch") -> ("Refname"=w202:string)
        n102 = call "DBToString.vi"("Enum"=DBNameEnum."QSWaitBeforeFire") -> ("Refname"=w153:string)
        n103 = call "DBToString.vi"("Enum"=DBNameEnum."QSWaitBeforeRetract") -> ("Refname"=w150:string)
        n104 = call "DBToString.vi"("Enum"=DBNameEnum."AngleBackwardValue") -> ("Refname"=w144:string)
        n105 = call "DBToString.vi"("Enum"=DBNameEnum."AngleForwardValue") -> ("Refname"=w147:string)
        n106 = call <vilib>:"SD Write Number.vi"("Numeric"="InitialWait (ms)", "Name"=w203) -> ()  [unwired: 8 in, 2 out]
        n107 = call <vilib>:"SD Write Number.vi"("Numeric"="WaitBetweenLaunch (ms)", "Name"=w202) -> ()  [unwired: 8 in, 2 out]
        n108 = call <vilib>:"SD Write Number.vi"("Numeric"="HalfSpeedFactor", "Name"=w131) -> ()  [unwired: 8 in, 2 out]
        n109 = call <vilib>:"SD Write Number.vi"("Numeric"="QSWaitBeforeRetract (ms)", "Name"=w150) -> ()  [unwired: 8 in, 2 out]
        n110 = call <vilib>:"SD Write Number.vi"("Numeric"="QSWaitBeforeFire (ms)", "Name"=w153) -> ()  [unwired: 8 in, 2 out]
        n111 = call <vilib>:"SD Write Number.vi"("Numeric"="AngleForwardValue", "Name"=w147) -> ()  [unwired: 8 in, 2 out]
        n112 = call <vilib>:"SD Write Number.vi"("Numeric"="AngleBackwardValue", "Name"=w144) -> ()  [unwired: 8 in, 2 out]
        n113 = disable-structure shown="Enabled" {
          frame Enabled {
            n114 = call "DBToString.vi"("Enum"=DBNameEnum."UseAngleEncoder") -> ("Refname"=w242:string)
            n115 = call "DBToString.vi"("Enum"=DBNameEnum."UseLauncherPID") -> ("Refname"=w237:string)
            n116 = call "DBToString.vi"("Enum"=DBNameEnum."UseLauncherEncoder") -> ("Refname"=w238:string)
            n117 = call <vilib>:"SD Write Boolean.vi"("Boolean"="UseAngleEncoder", "Name"=w242) -> ()  [unwired: 8 in, 2 out]
            n118 = call <vilib>:"SD Write Boolean.vi"("Boolean"="UseLauncherPID", "Name"=w237) -> ()  [unwired: 8 in, 2 out]
            n119 = call <vilib>:"SD Write Boolean.vi"("Boolean"="UseLauncherEncoder", "Name"=w238) -> ()  [unwired: 8 in, 2 out]
          }
          frame Disabled {
          }
        }
        n120 = call "DBToString.vi"("Enum"=DBNameEnum."RPMPresets") -> ("Refname"=w198:string)
        n121 = Flatten To String(anything="RPMPresets") -> (data string=w222:string)  [unwired: 3 in, 2 out]
        n122 = call "DBToString.vi"("Enum"=DBNameEnum."AnglePresets") -> ("Refname"=w197:string)
        n123 = Flatten To String(anything="AnglePresets") -> (data string=w223:string)  [unwired: 3 in, 2 out]
        n124 = call <vilib>:"SD Write String.vi"("String"=w222, "Name"=w198) -> ()  [unwired: 8 in, 2 out]
        n125 = call <vilib>:"SD Write String.vi"("String"=w223, "Name"=w197) -> ()  [unwired: 8 in, 2 out]
      }
    }
  }
  n126 = while {
    tunnel: w44 -> [w251]
    tunnel: w40 -> [w248]
    tunnel: [w246] -> _
    i -> [w246]
    stop <- FALSE stop-if-true
    n127 = Wait on Notification(notifier=w248) -> (notification=w247:string, timed out?=w249:bool)  [unwired: 3 in, 2 out]
    n128 = case shown="False" w249 {
      tunnel: w251 -> [w253 _]
      tunnel: w247 -> [w252 _]
      frame False {
        n129 = call <vilib>:"Bind Controls to SmartDashboard.vi"("Bound Control Refs"=w253, "Server IP Address"=w252) -> ()  [unwired: 10 in]
      }
      frame True {
      }
    }
  }
  n130 = call "Get All Users Directory.vi"() -> ("All User Path"=w26:path)
  n131 = Build Path(base path=w26, name or relative path=path "Documents/FRC/DashboardSettings.ini") -> (appended path=w25:path)
  n132 = Build Path(base path=w26, name or relative path=path "Documents/FRC/Checklist.txt") -> (appended path=w30:path)
  n133 = call <vilib>:"Open Config Data.vi"("configuration file path"=w25) -> ("refnum"=w24:T21)  [unwired: 8 in, 2 out]
  n134 = call-poly <vilib>:"Read Key.vi"("section"=w21, "default value"="320x240", "key"="Size", "refnum"=w24) -> ("value"=w11:string, "refnum out"=w6:T21)  [unwired: 2 in, 4 out]
  n135 = Read from Text File(file (use dialog)=w30, count=-1 ("timeout ms (25000)")) -> (refnum out=w8:refnum<file>, text=w31:string[], error out=w32:errorcluster)  [unwired: 2 in, 1 out]
  n136 = case shown="Error" w32 {
    tunnel: w31 -> [w255 _]
    tunnel: [w255 w257] -> w28
    tunnel: w29 -> [_ w257]
    tunnel: w30 -> [_ w258]
    tunnel: [w254 w256] -> w7
    tunnel: w8 -> [w254 _]
    frame No Error {
    }
    frame Error {
      n137 = Write to Text File(file (use dialog)=w258, text=w257) -> (refnum out=w256:refnum<file>)  [unwired: 2 in, 2 out]
    }
  }
  n138 = call-poly <vilib>:"Read Key.vi"("section"=w21, "default value"=30, "key"="FrameRate", "refnum"=w6) -> ("value"=w16:i32, "refnum out"=w5:T21)  [unwired: 1 in, 5 out]
  n139 = control-ref of="Tree"() -> (w2:refnum<vi>)
  n140 = property on="Listbox" class="LstBox (strict)"("Item Symbols"=i32[] [], "Item Names"=w28) -> ()  [unwired: 2 in, 2 out]
  n141 = Close File(refnum=w7) -> ()  [unwired: 1 in, 2 out]
  n142 = call-poly <vilib>:"Read Key.vi"("section"=w21, "default value"=30, "key"="Compression", "refnum"=w5) -> ("value"=w15:i32, "refnum out"=w3:T21)  [unwired: 1 in, 5 out]
  n143 = while {
    tunnel: [w260] -> _
    tunnel: w2 -> [w259]
    i -> [w260]
    stop <- FALSE stop-if-true
    n144 = Wait (ms)(milliseconds to wait=u32 60) -> ()  [unwired: 1 out]
    n145 = case shown="\"Variables\"" "Viewer" {
      tunnel: w259 -> [_ w264]
      frame Default {
      }
      frame "Variables" {
        n146 = call <vilib>:"NT Read and Format Entries as Tree.vi"("Tree Refnum"=w264) -> ()  [unwired: 9 in, 2 out]
      }
    }
  }
  n147 = control-ref of="Test Tree"() -> (w1:refnum<vi>)
  n148 = while {
    tunnel: w13 -> [w269]
    shift-right: [w268] -> _
    shift-left: w3 -> [w267]
    tunnel: [w266] -> _
    tunnel: w1 -> [w265]
    i -> [w266]
    stop <- FALSE stop-if-true
    (unwired) 0.0 ("Meter")
    n149 = event shown="[0] Timeout" {
      selector: _ -> [_ _ _ _ _ _ _ _ _ _ _ _ _]
      dyn-events: _ -> [_ _ _ _ _ _ _ _ _ _ _ _ _]
      timeout: u32 60 ("milliseconds to wait") -> [_ _ _ _ _ _ _ _ _ _ _ _ _]
      tunnel: w265 -> [w279 _ _ _ _ _ _ _ _ _ _ _ _]
      tunnel: "Test Tree" -> [_ _ _ _ _ _ _ _ w473 w481 w483 w487 w495]
      tunnel: w269 -> [_ w301 _ _ _ _ w437 w467 _ _ _ _ _]
      tunnel: [w273 w300 _ w403 w411 w423 w436 w460 w472 w479 w482 w486 w494] -> w268
      tunnel: w267 -> [w273 w300 _ w403 w411 w423 w435 w460 w472 w479 w482 w486 w494]
      event Timeout {
        w278 = enum16{"Update", "Clear"}[] [enum."Clear", enum."Clear", enum."Clear", enum."Clear", enum."Update", enum."Update", enum."Clear"] items=["Update", "Clear"]
        n150 = event-data() -> ()  [unwired: 1 in, 1 out]
        n151 = local read "Mode"() -> (w276:T2)
        n152 = Index Array(array=w278, index=w276) -> (element=w277:enum16{"Update", "Clear"})
        n153 = call <vilib>:"NT Read String.vi"("Name"="TestMode/TestName") -> ("String"=w282:string)  [unwired: 9 in, 1 out]
        n154 = case shown="\"Ops\", Default" "Dashboard Tab" {
          tunnel: w279 -> [_ w292]
          tunnel: "/TestMode/Automatic/" ("Name Pattern") -> [_ w291]
          tunnel: w277 -> [_ w290]
          tunnel: w276 -> [_ w288]
          frame "Ops", Default {
          }
          frame "Test" {
            w287 = -2 ("Active Item:Row Number")
            n155 = call <vilib>:"NT Read and Format Entries as Tree.vi"("Operation"=w290, "Name Pattern"=w291, "Tree Refnum"=w292) -> ()  [unwired: 7 in, 2 out]
            n156 = Index Array(array=u32[] [14013909, 14013909, 14013909, 14013909, 14013909, 16777215, 14013909], index=w288) -> (element=w286:u32)
            n157 = property on="Test Tree" class="Tree (strict)"("Active Item Row Number"=w287, "ActiveColNum"=w287, "CellBG"=w286, "Active Item Row Number"=-1 ("Active Item:Row Number"), "CellBG"=u32 5789784 ("Color Box")) -> ()  [unwired: 2 in, 2 out]
          }
        }
        n158 = case shown="\"\"" w282 {
          tunnel: "TestMode/TestProgress" ("Name") -> [w294 _]
          tunnel: "TestMode/TestProgressText" ("Name") -> [w293 _]
          frame Default {
            n159 = call <vilib>:"NT Read Number.vi"("Name"=w294) -> ("Numeric"=w295:dbl)  [unwired: 9 in, 1 out]
            n160 = call <vilib>:"NT Read String.vi"("Name"=w293) -> ("String"=w296:string)  [unwired: 9 in, 1 out]
            n161 = Bundle("Numeric"=w295, "String"=w296) -> (→"Progress":cluster{"Numeric":dbl, "String":string})  [unwired: 1 in]
          }
          frame "" {
            n162 = property on="Progress" class="Clust (strict)"("Visible"=FALSE) -> ()  [unwired: 2 in, 2 out]
            n163 = local write "Test Name"(u16 0) -> ()
          }
        }
      }
      event "Test Tree": Value Change {
        # "Show appropriate\ncontrols"
        n164 = event-data() -> ("CtlRef"=w304:refnum<vi>, "NewVal"=w302:string)  [unwired: 1 in]
        n165 = call <vilib>:"WPI_UtilitiesGetTreeIOName.vi"("NewVal"=w302, "TreeControl in"=w304) -> ("I/O Name"=w305:string)  [unwired: 9 in]
        n166 = case shown="\"Camera\"" w305 {
          selector: w305 -> [_ w312 _ w330 w339 _]
          tunnel: w302 -> [_ _ w327 w329 _ w346]
          tunnel: w301 -> [_ _ _ _ _ w345]
          frame Default {
            w307 = FALSE ("Visible")
            w306 = FALSE ("Visible")
            n167 = property on="Motor" class="Clust (strict)"("Visible"=w306) -> ()  [unwired: 2 in, 2 out]
            n168 = property on="Ring" class="Ring (strict)"("Visible"=w306) -> ()  [unwired: 2 in, 2 out]
            n169 = property on="Rev/Fwd" class="Clust (strict)"("Visible"=w307) -> ()  [unwired: 2 in, 2 out]
            n170 = property on="On/Off" class="Bool (strict)"("Visible"=w307) -> ()  [unwired: 2 in, 2 out]
            n171 = property on="Slider" class="Slide (strict)"("Visible"=w307) -> ()  [unwired: 2 in, 2 out]
          }
          frame "Motor", "PWM" {
            w313 = FALSE ("Visible")
            n172 = case shown="\"Motor\", Default" w312 {
              tunnel: [1.0 ("Value") -1.0 ("Value")] -> w311
              tunnel: [255.0 ("Value") 1.0 ("Value")] -> w310
              tunnel: [128.0 ("Value") 0.0 ("Value")] -> w309
              tunnel: [64.0 ("Value") 0.5 ("Value")] -> w308
              frame "PWM" {
              }
              frame "Motor", Default {
              }
            }
            n173 = property on="Motor" class="Clust (strict)"("Visible"=TRUE) -> ()  [unwired: 2 in, 2 out]
            n174 = property on="Value" class="Slide (strict)"("Value"=w309, "Scale.Minimum"=w311, "Scale.Maximum"=w310, "Scale.Increment"=w308) -> ()  [unwired: 2 in, 2 out]
            n175 = property on="On/Off" class="Bool (strict)"("Visible"=w313) -> ()  [unwired: 2 in, 2 out]
            n176 = property on="Slider" class="Slide (strict)"("Visible"=w313) -> ()  [unwired: 2 in, 2 out]
            n177 = property on="Ring" class="Ring (strict)"("Visible"=w313) -> ()  [unwired: 2 in, 2 out]
            n178 = property on="Rev/Fwd" class="Clust (strict)"("Visible"=w313) -> ()  [unwired: 2 in, 2 out]
          }
          frame "Servo" {
            w325 = FALSE ("Visible")
            n179 = call <vilib>:"NT Read Number.vi"("Name"=w327) -> ("Numeric"=w326:dbl)  [unwired: 9 in, 1 out]
            n180 = property on="Slider" class="Slide (strict)"("Visible"=TRUE, "Scale.Maximum"=170.0 ("Scale.Range:Maximum")) -> ()  [unwired: 2 in, 2 out]
            n181 = local write "Slider"(w326) -> ()
            n182 = property on="Motor" class="Clust (strict)"("Visible"=w325) -> ()  [unwired: 2 in, 2 out]
            n183 = property on="Rev/Fwd" class="Clust (strict)"("Visible"=w325) -> ()  [unwired: 2 in, 2 out]
            n184 = property on="On/Off" class="Bool (strict)"("Visible"=w325) -> ()  [unwired: 2 in, 2 out]
            n185 = property on="Ring" class="Ring (strict)"("Visible"=w325) -> ()  [unwired: 2 in, 2 out]
          }
          frame "Relay", "Solenoid" {
            w328 = FALSE ("Visible")
            n186 = property on="Motor" class="Clust (strict)"("Visible"=w328) -> ()  [unwired: 2 in, 2 out]
            n187 = property on="Slider" class="Slide (strict)"("Visible"=w328) -> ()  [unwired: 2 in, 2 out]
            n188 = Search and Replace String(input string=w329, search string="/Value  **", replace string="/Direction") -> (result string=w335:string)  [unwired: 5 in, 3 out]
            n189 = property on="Ring" class="Ring (strict)"("Visible"=w328) -> ()  [unwired: 2 in, 2 out]
            n190 = call <vilib>:"NT Read String.vi"("Name"=w335) -> ("String"=w333:string)  [unwired: 9 in, 1 out]
            n191 = Equal?(x="Both directions", y=w333) -> (x = y?=w331:bool)
            n192 = Not(x=w331) -> (.not. x?=w332:bool)
            n193 = property on="Rev/Fwd" class="Clust (strict)"("Visible"=w331) -> ()  [unwired: 2 in, 2 out]
            n194 = property on="On/Off" class="Bool (strict)"("Visible"=w332, "Caption.Text"=w330) -> ()  [unwired: 2 in, 2 out]
          }
          frame "Compressor", "Digital Out" {
            w338 = FALSE ("Visible")
            # "Get direction and finish"
            n195 = property on="Motor" class="Clust (strict)"("Visible"=w338) -> ()  [unwired: 2 in, 2 out]
            n196 = property on="Slider" class="Slide (strict)"("Visible"=w338) -> ()  [unwired: 2 in, 2 out]
            n197 = property on="Ring" class="Ring (strict)"("Visible"=w338) -> ()  [unwired: 2 in, 2 out]
            n198 = property on="On/Off" class="Bool (strict)"("Visible"=TRUE, "Caption.Text"=w339) -> ()  [unwired: 2 in, 2 out]
            n199 = property on="Rev/Fwd" class="Clust (strict)"("Visible"=FALSE) -> ()  [unwired: 2 in, 2 out]
          }
          frame "Camera" {
            n200 = call <vilib>:"Get Last Path Segment.vi"("String in"=w346) -> ("String out"=w347:string)  [unwired: 10 in]
            n201 = property on="On/Off" class="Bool (strict)"("Visible"=FALSE) -> ()  [unwired: 2 in, 2 out]
            n202 = property on="Motor" class="Clust (strict)"("Visible"=FALSE) -> ()  [unwired: 2 in, 2 out]
            n203 = property on="Rev/Fwd" class="Clust (strict)"("Visible"=FALSE) -> ()  [unwired: 2 in, 2 out]
            n204 = case shown="\"White Balance  **\"" w347 {
              tunnel: w346 -> [w353 w362 w371 w380 w389 _ w395]
              tunnel: w345 -> [w351 w359 w368 w377 w386 _ _]
              frame "Size  **" {
                n205 = Index Array(array=w351) -> (element=w350:cluster{string[]})  [unwired: 1 in]
                n206 = call <vilib>:"NT Read String.vi"("Name"=w353) -> ("String"=w352:string)  [unwired: 9 in, 1 out]
                n207 = Unbundle(w350) -> (w348:string[])
                n208 = Match First String(2:w348, 3:w352) -> (0:w349:i32)  [unwired: 1 out]
                n209 = property on="Ring" class="Ring (strict)"("Value"=w349, "Strings []"=w348) -> ()  [unwired: 2 in, 2 out]
                n210 = property on="Ring" class="Ring (strict)"("Visible"=TRUE) -> ()  [unwired: 2 in, 2 out]
                n211 = property on="Slider" class="Slide (strict)"("Visible"=FALSE) -> ()  [unwired: 2 in, 2 out]
              }
              frame "White Balance  **" {
                n212 = Index Array(array=w359, index=1) -> (element=w360:cluster{string[]})
                n213 = call <vilib>:"NT Read String.vi"("Name"=w362) -> ("String"=w361:string)  [unwired: 9 in, 1 out]
                n214 = Unbundle(w360) -> (w357:string[])
                n215 = Match First String(2:w357, 3:w361) -> (0:w356:i32)  [unwired: 1 out]
                n216 = property on="Ring" class="Ring (strict)"("Value"=w356, "Strings []"=w357) -> ()  [unwired: 2 in, 2 out]
                n217 = property on="Ring" class="Ring (strict)"("Visible"=TRUE) -> ()  [unwired: 2 in, 2 out]
                n218 = property on="Slider" class="Slide (strict)"("Visible"=FALSE) -> ()  [unwired: 2 in, 2 out]
              }
              frame "Exposure  **" {
                n219 = Index Array(array=w368, index=2) -> (element=w369:cluster{string[]})
                n220 = call <vilib>:"NT Read String.vi"("Name"=w371) -> ("String"=w370:string)  [unwired: 9 in, 1 out]
                n221 = Unbundle(w369) -> (w365:string[])
                n222 = Match First String(2:w365, 3:w370) -> (0:w366:i32)  [unwired: 1 out]
                n223 = property on="Ring" class="Ring (strict)"("Value"=w366, "Strings []"=w365) -> ()  [unwired: 2 in, 2 out]
                n224 = property on="Ring" class="Ring (strict)"("Visible"=TRUE) -> ()  [unwired: 2 in, 2 out]
                n225 = property on="Slider" class="Slide (strict)"("Visible"=FALSE) -> ()  [unwired: 2 in, 2 out]
              }
              frame "Exposure Priority  **" {
                n226 = Index Array(array=w377, index=3) -> (element=w378:cluster{string[]})
                n227 = call <vilib>:"NT Read String.vi"("Name"=w380) -> ("String"=w379:string)  [unwired: 9 in, 1 out]
                n228 = Unbundle(w378) -> (w374:string[])
                n229 = Match First String(2:w374, 3:w379) -> (0:w375:i32)  [unwired: 1 out]
                n230 = property on="Ring" class="Ring (strict)"("Value"=w375, "Strings []"=w374) -> ()  [unwired: 2 in, 2 out]
                n231 = property on="Ring" class="Ring (strict)"("Visible"=TRUE) -> ()  [unwired: 2 in, 2 out]
                n232 = property on="Slider" class="Slide (strict)"("Visible"=FALSE) -> ()  [unwired: 2 in, 2 out]
              }
              frame "Color Enable  **" {
                n233 = Index Array(array=w386, index=4) -> (element=w387:cluster{string[]})
                n234 = call <vilib>:"NT Read String.vi"("Name"=w389) -> ("String"=w388:string)  [unwired: 9 in, 1 out]
                n235 = Unbundle(w387) -> (w383:string[])
                n236 = Match First String(2:w383, 3:w388) -> (0:w384:i32)  [unwired: 1 out]
                n237 = property on="Ring" class="Ring (strict)"("Value"=w384, "Strings []"=w383) -> ()  [unwired: 2 in, 2 out]
                n238 = property on="Ring" class="Ring (strict)"("Visible"=TRUE) -> ()  [unwired: 2 in, 2 out]
                n239 = property on="Slider" class="Slide (strict)"("Visible"=FALSE) -> ()  [unwired: 2 in, 2 out]
              }
              frame Default {
                n240 = property on="Ring" class="Ring (strict)"("Visible"=FALSE) -> ()  [unwired: 2 in, 2 out]
                n241 = property on="Slider" class="Slide (strict)"("Visible"=FALSE) -> ()  [unwired: 2 in, 2 out]
              }
              frame "Brightness  **", "Color Level  **", "Compression  **", "FPS  **", "Sharpness  **" {
                n242 = call <vilib>:"NT Read Number.vi"("Name"=w395) -> ("Numeric"=w394:dbl)  [unwired: 9 in, 1 out]
                n243 = local write "Slider"(w394) -> ()
                n244 = property on="Slider" class="Slide (strict)"("Visible"=TRUE, "Scale.Maximum"=100.0 ("Scale.Range:Maximum")) -> ()  [unwired: 2 in, 2 out]
                n245 = property on="Ring" class="Ring (strict)"("Visible"=FALSE) -> ()  [unwired: 2 in, 2 out]
              }
            }
          }
        }
        n246 = property on="Progress" class="Clust (strict)"("Visible"=FALSE) -> ()  [unwired: 2 in, 2 out]
      }
      event "Test Name": Mouse Enter {
        # "Populate the ring with the list of tests"
        n247 = event-data() -> ()  [unwired: 1 in, 1 out]
        n248 = call <vilib>:"NT Read String Array.vi"("Name"="TestMode/TestList") -> ("String Array"=w402:string[])  [unwired: 9 in, 1 out]
        n249 = Build Array (concatenate)("Select the test to run...", w402) -> (w401:string[])
        n250 = property on="Test Name" class="Ring (strict)"("Strings []"=w401) -> ()  [unwired: 2 in, 2 out]
      }
      event "Test Name": Value Change {
        w404 = FALSE ("Visible")
        # "Tell the robot the test name to run"
        n251 = event-data() -> ("NewVal"=w408:u16)  [unwired: 1 in]
        n252 = property on="Test Name" class="Ring (strict)"() -> ("Strings []"=w409:string[])  [unwired: 2 in, 2 out]
        n253 = local write "Progress"(T8 {"Test Progress"=0, "Test Progress Text"=""} ("Progress")) -> ()
        n254 = Index Array(array=w409, index=w408) -> (element=w407:string)
        n255 = call <vilib>:"NT Write String.vi"("String"=w407, "Name"="TestMode/TestName") -> ()  [unwired: 9 in, 1 out]
        n256 = property on="Progress" class="Clust (strict)"("Visible"=TRUE) -> ()  [unwired: 2 in, 2 out]
        n257 = property on="Motor" class="Clust (strict)"("Visible"=w404) -> ()  [unwired: 2 in, 2 out]
        n258 = property on="Slider" class="Slide (strict)"("Visible"=w404) -> ()  [unwired: 2 in, 2 out]
        n259 = property on="On/Off" class="Bool (strict)"("Visible"=w404) -> ()  [unwired: 2 in, 2 out]
        n260 = property on="Rev/Fwd" class="Clust (strict)"("Visible"=w404) -> ()  [unwired: 2 in, 2 out]
        n261 = property on="Ring" class="Ring (strict)"("Visible"=w404) -> ()  [unwired: 2 in, 2 out]
      }
      event "Listbox": Double Click {
        n262 = event-data() -> ("PlatMods.Shift"=w412:bool, "Row"=w414:i32)  [unwired: 1 in]
        n263 = case shown="False" w412 {
          tunnel: w414 -> [w418 _]
          tunnel: 1 -> [w417 _]
          frame False {
            n264 = property on="Listbox" class="LstBox (strict)"() -> ("Item Symbols"=w416:i32[])  [unwired: 2 in, 2 out]
            n265 = Replace Array Subset(array=w416, new element=w417, index=w418) -> (w415:i32[])
            n266 = property on="Listbox" class="LstBox (strict)"("Item Symbols"=w415) -> ()  [unwired: 2 in, 2 out]
          }
          frame True {
            w419 = 0 ("Top Row")
            n267 = property on="Listbox" class="LstBox (strict)"() -> ("Number of Rows"=w421:u32)  [unwired: 2 in, 2 out]
            n268 = Initialize Array(0, w421) -> (w420:i32[])
            n269 = property on="Listbox" class="LstBox (strict)"("Top Row"=w419, "Value"=w419, "Item Symbols"=w420) -> ()  [unwired: 2 in, 2 out]
          }
        }
      }
      event "Listbox": Key Down {
        n270 = event-data() -> ("VKey"=w425:T22)  [unwired: 1 in]
        n271 = case shown="\"Left\", \"Right\"" w425 {
          selector: w425 -> [w430 _]
          tunnel: eventvkey."Left" ("VKey") -> [w428 _]
          frame "Left", "Right" {
            n272 = Equal?(x=w428, y=w430) -> (x = y?=w429:bool)
            n273 = Select(t=0, s=w429, f=1) -> (s? t:f=w431:i32)
            n274 = property on="Listbox" class="LstBox (strict)"() -> ("Item Symbols"=w434:i32[])  [unwired: 2 in, 2 out]
            n275 = Replace Array Subset(array=w434, new element=w431, index="Listbox") -> (w433:i32[])
            n276 = property on="Listbox" class="LstBox (strict)"("Item Symbols"=w433) -> ()  [unwired: 2 in, 2 out]
          }
          frame Default {
          }
        }
      }
      event "DB Camera Config": Value Change {
        n277 = event-data() -> ("NewVal"=w438:bool)  [unwired: 1 in]
        n278 = case shown="False" w438 {
          tunnel: w437 -> [w447 _]
          tunnel: [w440 w458] -> w436
          tunnel: w435 -> [w439 w458]
          frame False {
            w454 = "Camera"
            w457 = FALSE ("Visible")
            n279 = local read "Camera Settings"() -> (w446:T1)
            n280 = Index Array(array=w447) -> (element=w450:cluster{string[]})  [unwired: 1 in]
            n281 = Unbundle(w446) -> ("Frate Rate"=w445:i32, "Compression"=w444:i32, "Size"=w448:u16)
            n282 = Unbundle(w450) -> (w449:string[])
            n283 = Index Array(array=w449, index=w448) -> (element=w443:string)
            n284 = call-poly <vilib>:"Write Key.vi"("section"=w454, "value"=w443, "key"="Size", "refnum"=w439) -> ("refnum out"=w456:T21)  [unwired: 2 in, 5 out]
            n285 = call-poly <vilib>:"Write Key.vi"("section"=w454, "value"=w445, "key"="FrameRate", "refnum"=w456) -> ("refnum out"=w455:T21)  [unwired: 1 in, 6 out]
            n286 = property on="Camera Settings" class="Clust (strict)"("Visible"=w457) -> ()  [unwired: 2 in, 2 out]
            n287 = local write "DB Camera Config"(w457) -> ()
            n288 = call-poly <vilib>:"Write Key.vi"("section"=w454, "value"=w444, "key"="Compression", "refnum"=w455) -> ("refnum out"=w441:T21)  [unwired: 1 in, 6 out]
            n289 = call <vilib>:"Close Config Data.vi"("refnum"=w441) -> ("file path"=w442:path)  [unwired: 2 in, 8 out]
            n290 = call <vilib>:"Open Config Data.vi"("configuration file path"=w442) -> ("refnum"=w440:T21)  [unwired: 8 in, 2 out]
          }
          frame True {
            n291 = property on="Camera Settings" class="Clust (strict)"("Visible"=TRUE) -> ()  [unwired: 2 in, 2 out]
          }
        }
      }
      event "Camera Settings": Value Change {
        n292 = event-data() -> ("NewVal"=w471:T1)  [unwired: 1 in]
        n293 = Index Array(array=w467) -> (element=w466:cluster{string[]})  [unwired: 1 in]
        n294 = Unbundle(w471) -> ("Frate Rate"=w462:i32, "Compression"=w461:i32, "Size"=w464:u16)
        n295 = Unbundle(w466) -> (w465:string[])
        n296 = Index Array(array=w465, index=w464) -> (element=w463:string)
        n297 = Format Into String(format string="%s   %dfps   %d%%", w463, w462, w461) -> (resulting string=w468:string)  [unwired: 2 in, 1 out]
        n298 = Build Array(w468) -> (w469:string[])
        n299 = property on="DB Camera Config" class="Bool (strict)"("Strings [4]"=w469) -> ()  [unwired: 2 in, 2 out]
      }
      event "Motor.Enable": Value Change {
        n300 = event-data() -> ("NewVal"=w477:bool)  [unwired: 1 in]
        n301 = Unbundle("Motor") -> ("Value"=w476:dbl)  [unwired: 1 out]
        n302 = Select(t=w476, s=w477, f=0.0) -> (s? t:f=w474:dbl)
        n303 = call <vilib>:"NT Write Number.vi"("Numeric"=w474, "Name"=w473) -> ()  [unwired: 9 in, 1 out]
      }
      event "Slider": Value Change {
        n304 = event-data() -> ("NewVal"=w480:dbl)  [unwired: 1 in]
        n305 = call <vilib>:"NT Write Number.vi"("Numeric"=w480, "Name"=w481) -> ()  [unwired: 9 in, 1 out]
      }
      event "On/Off": Value Change {
        n306 = event-data() -> ("NewVal"=w485:bool)  [unwired: 1 in]
        n307 = Boolean To (0,1)(Boolean=w485) -> (0, 1=w484:i16)
        n308 = call <vilib>:"NT Write Number.vi"("Numeric"=w484, "Name"=w483) -> ()  [unwired: 9 in, 1 out]
      }
      event "Rev/Fwd": Value Change {
        n309 = event-data() -> ("NewVal.Forward"=w493:bool, "NewVal.Reverse"=w492:bool)  [unwired: 1 in]
        n310 = Boolean To (0,1)(Boolean=w493) -> (0, 1=w489:i16)
        n311 = Boolean To (0,1)(Boolean=w492) -> (0, 1=w491:i16)
        n312 = Negate(x=w491) -> (-x=w490:i16)
        n313 = Add(x=w489, y=w490) -> (x+y=w488:i16)
        n314 = call <vilib>:"NT Write Number.vi"("Numeric"=w488, "Name"=w487) -> ()  [unwired: 9 in, 1 out]
      }
      event "Ring": Value Change {
        n315 = event-data() -> ("NewVal"=w497:u16)  [unwired: 1 in]
        n316 = property on="Ring" class="Ring (strict)"() -> ("Strings []"=w498:string[])  [unwired: 2 in, 2 out]
        n317 = Index Array(array=w498, index=w497) -> (element=w496:string)
        n318 = call <vilib>:"NT Write String.vi"("String"=w496, "Name"=w495) -> ()  [unwired: 9 in, 1 out]
      }
    }
  }
  n319 = Index Array(array=w13) -> (element=w14:cluster{string[]})  [unwired: 1 in]
  n320 = Unbundle(w14) -> (w12:string[])
  n321 = Match First String(2:w12, 3:w11) -> (0:w10:i32)  [unwired: 1 out]
  n322 = Bundle("value"=w16, "value"=w15, "index"=w10) -> (w4:cluster{"value":i32, "value":i32, "index":i32})  [unwired: 1 out]
  n323 = property on="On/Off" class="Bool (strict)"("Visible"=w27) -> ()  [unwired: 2 in, 2 out]
  n324 = property on="Motor" class="Clust (strict)"("Visible"=w27) -> ()  [unwired: 2 in, 2 out]
  n325 = property on="Progress" class="Clust (strict)"("Visible"=w27) -> ()  [unwired: 2 in, 2 out]
  n326 = property on="Ring" class="Ring (strict)"("Visible"=w27) -> ()  [unwired: 2 in, 2 out]
  n327 = property on="Camera Settings" class="Clust (strict)"("Val(Sgnl)"=w4) -> ()  [unwired: 2 in, 2 out]
  n328 = property on="Rev/Fwd" class="Clust (strict)"("Visible"=w27) -> ()  [unwired: 2 in, 2 out]
  n329 = property on="Camera Settings" class="Clust (strict)"("Visible"=w27) -> ()  [unwired: 2 in, 2 out]
  n330 = local write "DB Camera Config"(w27) -> ()
